vi "MoveRobot.vi"(6 "Drive":bool, 7 "PWM Offset":dbl=0.9, 8 "Motor PWMs":T8, 9 "Max Duty Cycle":dbl=0.7, 10 "Translation Response":dbl, 11 "Spin Response":dbl) -> ()   [LabVIEW 2018]
uses:
  <vilib>/myRIO/Instrument Drivers/Onboard IO/PWM/typedefs/PWM Reference.ctl
  <vilib>/myRIO/Common/Instrument Driver Framework/Utilities/typedefs/myRIO Generic Hardware Reference.ctl
  <vilib>/myRIO/Common/Instrument Driver Framework/Utilities/typedefs/Hardware Version Enum.ctl
  <vilib>/myRIO/Common/Instrument Driver Framework/Utilities/typedefs/myRIO v1.0 Reference.ctl
  <vilib>/myRIO/Common/Instrument Driver Framework/Utilities/typedefs/Generic FPGA Reference.ctl
  <vilib>/myRIO/Common/Instrument Driver Framework/myRIO v1.0/PWM/typedefs/PWM Channels Enum.ctl
  <vilib>/myRIO/Instrument Drivers/Onboard IO/PWM/typedefs/PWM Configuration.ctl
  <vilib>/myRIO/Instrument Drivers/Onboard IO/PWM/PWM.lvlib
panel:
  out "LMot":dbl(slide) scale=-1.0..1.0
  out "RMot":dbl(slide) scale=-1.0..1.0
  # "MoveRobot.vi"
  # "The MoveRobot.vi sums the a rotational and translational response for the robot to generate \ntwo doubles between [-1,1] (LMot, and RMot) which are used to drive the robot in a bulldozer\ntrack type manner.   \n\nThe PWM offset is handed to the UpdateMotors_BulldozerDrive.vi to bias the duty cycles of teh wheels\ntowards movement.\n\nAdditionally, a boolean control, Drive, is included which zeros the inputs to Update Motors when false."
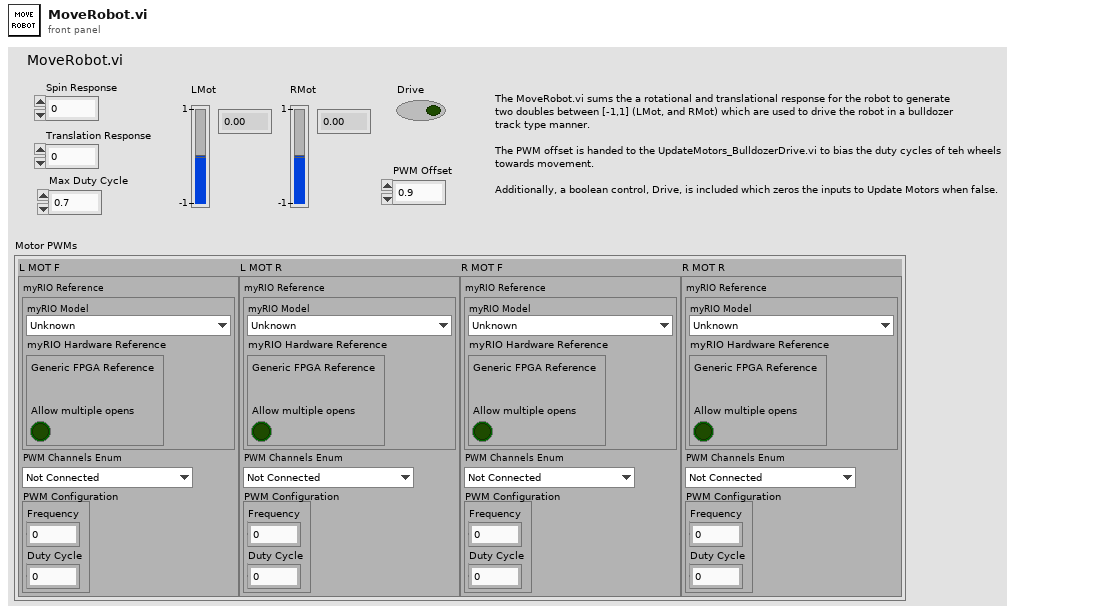
[diagram p1: front panel]
types:
  T1 = typedef "PWM.lvlib/PWM Reference.ctl" = cluster{"myRIO Reference":T2, "PWM Channels Enum":T6, "PWM Configuration":T7}
  T2 = typedef "myRIO Generic Hardware Reference.ctl" = cluster{"myRIO Model":T3, "myRIO Hardware Reference":T4}
  T3 = typedef "Hardware Version Enum.ctl" = enum16{"Unknown", "myRIO-1900", "myRIO-1950", "roboRIO", "NI ELVIS RIO CM", "ELVIS III"}
  T4 = typedef "myRIO v1.0 Reference.ctl" = cluster{"Generic FPGA Reference":T5, "Allow multiple opens":bool}
  T5 = typedef "Generic FPGA Reference.ctl" = refnum<k20>
  T6 = typedef "PWM Channels Enum.ctl" = enum16{"Not Connected", "C/PWM0", "C/PWM1", "A/PWM0", "A/PWM1", "A/PWM2", "A/PWM3", "A/PWM4", "A/PWM5", "A/PWM6", "A/PWM7", "A/PWM8", "A/PWM9", "A/PWM10", "A/PWM11", "A/PWM12", "A/PWM13", "A/PWM14", "A/PWM15", "A/PWM16", "A/PWM17", "A/PWM18", "A/PWM19", "B/PWM0", "B/PWM1", "B/PWM2", "B/PWM3", "B/PWM4", "B/PWM5", "B/PWM6", "B/PWM7", "B/PWM8", "B/PWM9", "B/PWM10", "B/PWM11", "B/PWM12", "B/PWM13", "B/PWM14", "B/PWM15", "B/PWM16", "B/PWM17", "B/PWM18", "B/PWM19", "PWM/PWM0", "PWM/PWM1", "PWM/PWM2", "PWM/PWM3", "PWM/PWM4", "PWM/PWM5", "PWM/PWM6", "PWM/PWM7", "PWM/PWM8", "PWM/PWM9"}
  T7 = typedef "PWM.lvlib/PWM Configuration.ctl" = cluster{"Frequency":dbl, "Duty Cycle":dbl}
  T8 = cluster{"L MOT F ":T1, "L MOT R":T1, "R MOT F":T1, "R MOT R":T1}
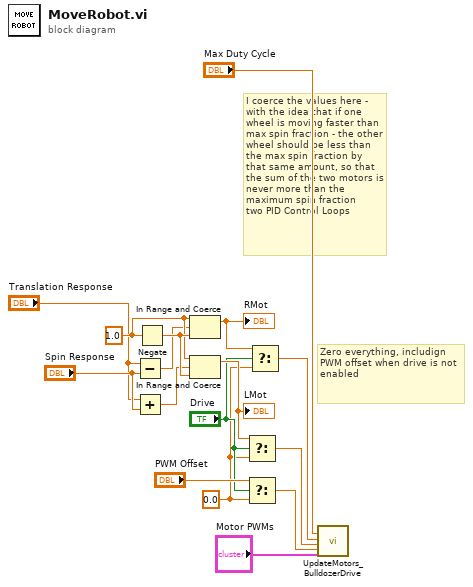
[diagram p0: block diagram]
diagram:
  w5 = 1.0
  w11 = 0.0 ("f")
  # "Zero everything, includign PWM offset when drive is not enabled"
  # "I coerce the values here - with the idea that if one wheel is moving faster than max spin fraction - the other wheel should be less than the max spin fraction by that same amount, so that the sum of the two motors is never more than the maximum spin fraction\ntwo PID Control Loops"
  n1 = Subtract(x="Translation Response", y="Spin Response") -> (x-y=w4:dbl)
  n2 = Add(x="Translation Response", y="Spin Response") -> (x+y=w1:dbl)
  n3 = Negate(x=w5) -> (-x=w16:dbl)
  n4 = In Range and Coerce(upper limit=w5, x=w4, lower limit=w16) -> (coerced(x)=w15:dbl)  [unwired: 1 out]
  "RMot" <- w15
  n5 = In Range and Coerce(upper limit=w5, x=w1, lower limit=w16) -> (coerced(x)=w14:dbl)  [unwired: 1 out]
  "LMot" <- w14
  n6 = Select(t=w14, s="Drive", f=w11) -> (s? t:f=w8:dbl)
  n7 = Select(t="PWM Offset", s="Drive", f=w11) -> (s? t:f=w7:dbl)
  n8 = Select(t=w15, s="Drive", f=w11) -> (s? t:f=w9:dbl)
  n9 = call "UpdateMotors_BulldozerDrive.vi"("Max Duty Cycle"="Max Duty Cycle", "RMot"=w9, "LMot"=w8, "PWM Offset"=w7, "Motor PWMs"="Motor PWMs") -> ()  [unwired: 15 in]
